vi "Match-Value Image (Greyscale).vi"(8 "error in (no error)":errorcluster, 9 "Value":u8, 10 "Match in":T1, 11 "Greyscale Image-Source":T1) -> (0 "error out":errorcluster, 3 "Match in (duplicate)":T1)   [LabVIEW 2020, in "g_ar_toolkit.image.lvlib"]
uses:
  g_ar_toolkit.image.lvlib
  Greyscale Image.ctl
  0720c4fc-c714-46e4-a6a5-fc7e731e80c2.vi
  g_ar_toolkit.common/Module Path.vi
  <vilib>/Utility/error.llb/Error Cluster From Error Code.vi
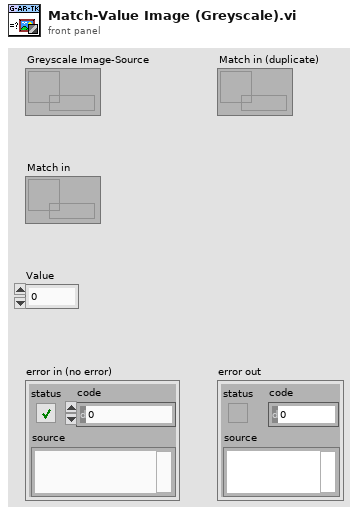
[diagram p1: front panel]
types:
  T1 = typedef "g_ar_toolkit.image.lvlib/Greyscale Image.ctl" = refnum<data-value>
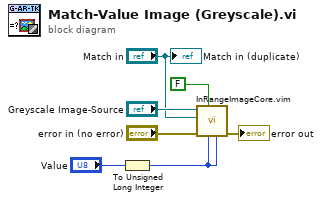
[diagram p0: block diagram]
diagram:
  n1 = To Unsigned Long Integer(number="Value") -> (unsigned 32bit integer=w1:u32)
  n2 = call "InRangeImageCore.vim"("Upper"=w1, "Lower"=w1, "IgnoreAlpha"=FALSE, "error in (no error)"="error in (no error)", "In-Range-Result"="Match in", "Src"="Greyscale Image-Source") -> ("error out"=→"error out":errorcluster)  [unwired: 5 in]
  "Match in (duplicate)" <- "Match in"
